vi "run_experiment_sCMOS_DAC.vi"() -> ()   [LabVIEW 2015]
uses:
  <vilib>/DAQmx/write.llb/DAQmx Write (Digital Bool 1Line 1Point).vi
  <vilib>/DAQmx/read.llb/DAQmx Read (Analog 1D Wfm NChan NSamp).vi
  <vilib>/DAQmx/read.llb/DAQmx Read (Digital 2D U32 NChan NSamp).vi
  <vilib>/DAQmx/write.llb/DAQmx Write (Digital 1D Wfm NChan NSamp).vi
  <vilib>/DAQmx/write.llb/DAQmx Write (Analog 1D DBL 1Chan NSamp).vi
  <vilib>/DAQmx/create/channels.llb/DAQmx Create Channel (DO-Digital Output).vi
  <vilib>/DAQmx/miscellaneous.llb/DAQmx Fill In Error Info.vi
  <vilib>/Utility/file.llb/Write Delimited Spreadsheet (DBL).vi
  <vilib>/Waveform/DWDTOps.llb/DWDT Uncompress Digital.vi
  <vilib>/addons/h5labview2/file/H5F.lvlib
panel:
  in  "New Session?":bool
  in  "New Session Type":enum32{"recording", "roi", "rig_state"}(radio)
  in  "Use Cam":bool
  in  "Pad Stim":bool
  out "Timestamp":string
  out "Genotype":string
  out "Fly Name":string
  out "Experiment Name":string
  out ".dcimg index":i32
  out ".dcimg count":i32
  in  "Use .dcimg":bool
  out "Cumulative Frames":i32
  out "N Stim Frames":i32
  out "Trial":i32
  out "N Samps 2 Write":i32
  out "AI/DI SampRate":dbl=1000.0 format="%0.2f"
  out "AO/DO SampRate":dbl
  out "DO Samps Written":u32
  out "AO Samps Written":u32
  out "Protocol Rate (Hz)":i32
  out "Num Stimuli":i32
  out "V Offset":i32
  out "H Offset":i32
  out "Rep":i32
  out ".dcimg --> .tiff":bool
  out "# tiffs":i32
  in  "Save .tiffs":bool
  in  "Configure Cam":bool
  out "Stimulus Order":i32[](array[numeric])
  in  "Randomize":bool
  out "Stop Input":bool
  out "temp .dcimg filepath":path
  out "Exposure":dbl
  out "V Width":i32
  out "H Width":i32
  out "Acquiring Frames":bool
  out "Current Stim Duration":dbl
  out "Current Stimulus Save Path":path
  in  "N Reps":dbl
  out "Experiment Path":path
  in  "Metadata Path":path
  out "Stimulus Files":path[](array[path])
  out "Protocol Name":string
  in  "Protocol Path":path
  out "Display":T1(plugin-control)
  out "DAC Input":waveform(dbl)[](graph) caption="DAC Input Display"
  out "error out":errorcluster
  out "Current Stimulus Name":string
  out "Curr Piezo Cmd":waveform(dbl)(graph)
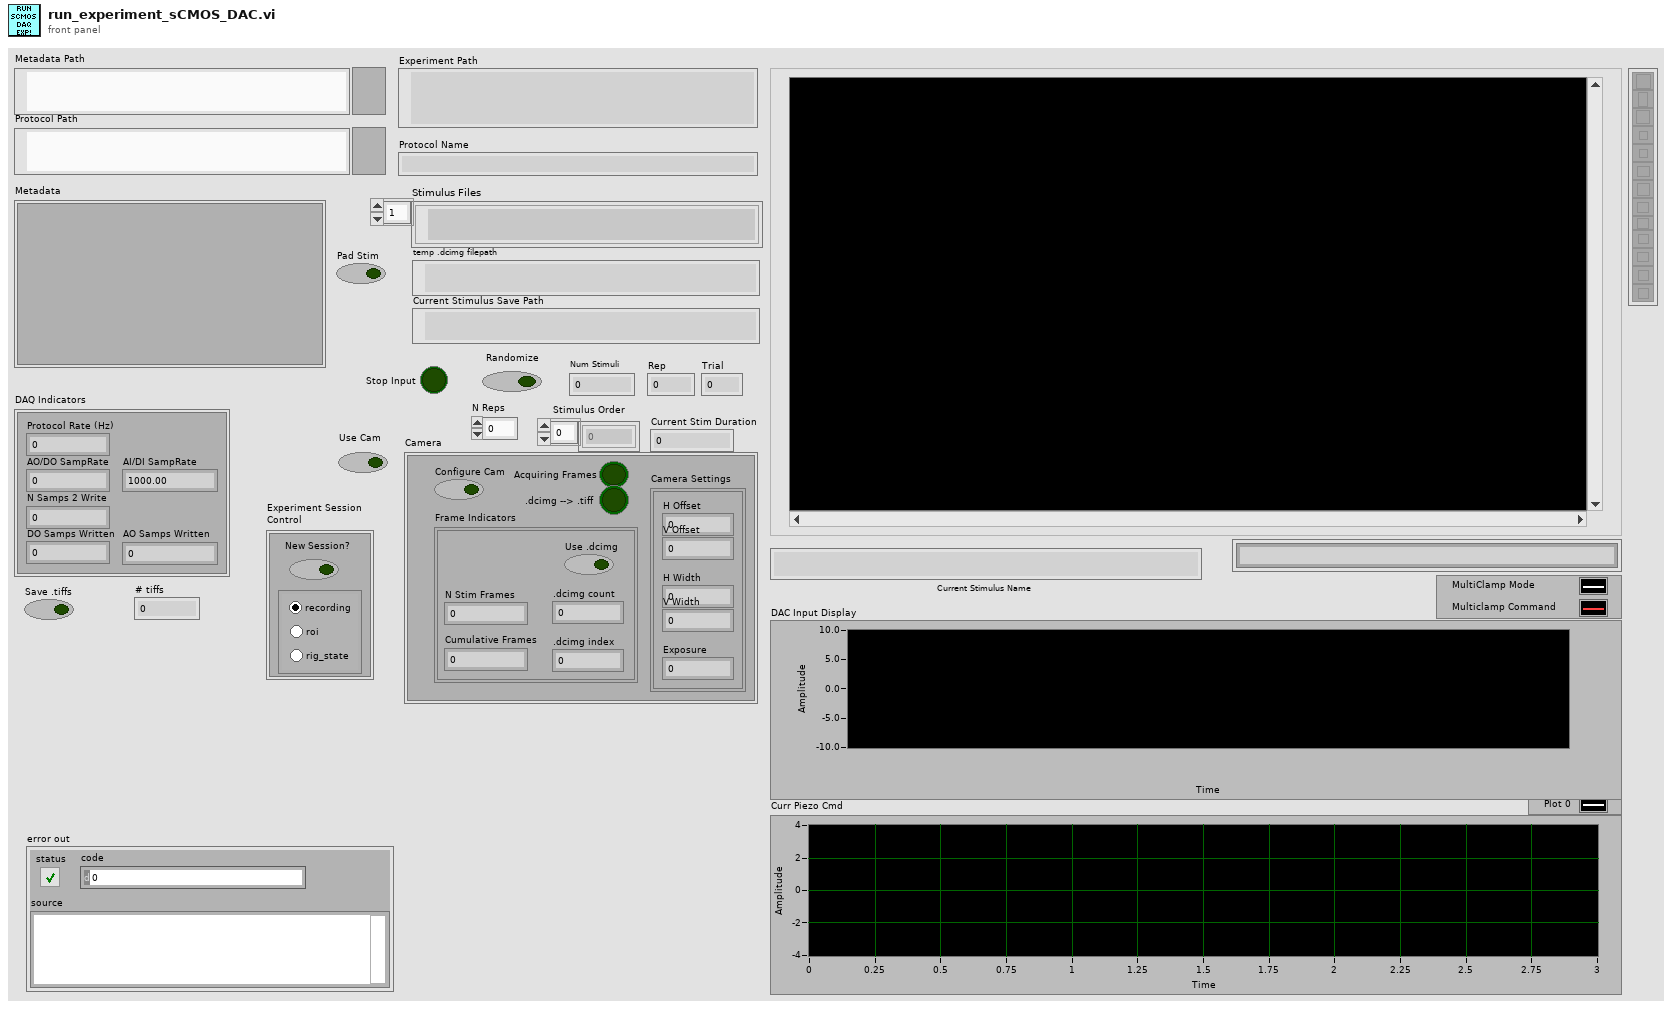
[diagram p1: front panel]
types:
  T1 = typedef "IMAQ Image.ctl" = refnum<image>
  T2 = cluster{"Value":i32, "Minimum":i32, "Maximum":i32, "Increment":i32}
  T3 = cluster{"Rows Per Strip":i32, "Photometric":i32, "Compression Type":i32}
  T4 = cluster{"piezo_command":dbl[], "alignment_command":dbl[]}
  T5 = typedef "Image Type" = u32
  T6 = cluster{"height":u32, "width":u32, "datatype":u32}
  T7 = cluster{"piezo_cmd":i32, "piezo_sensor":i32, "cam_trig_1":i32, "cam_trig_2":i32, "alignment_cmd":i32, "mc700b_primary":i32, "mc700b_secondary":i32, "mc700b_mode":i32, "mc700b_cmd":i32}
  T8 = typedef "hid_t.ctl" = i32
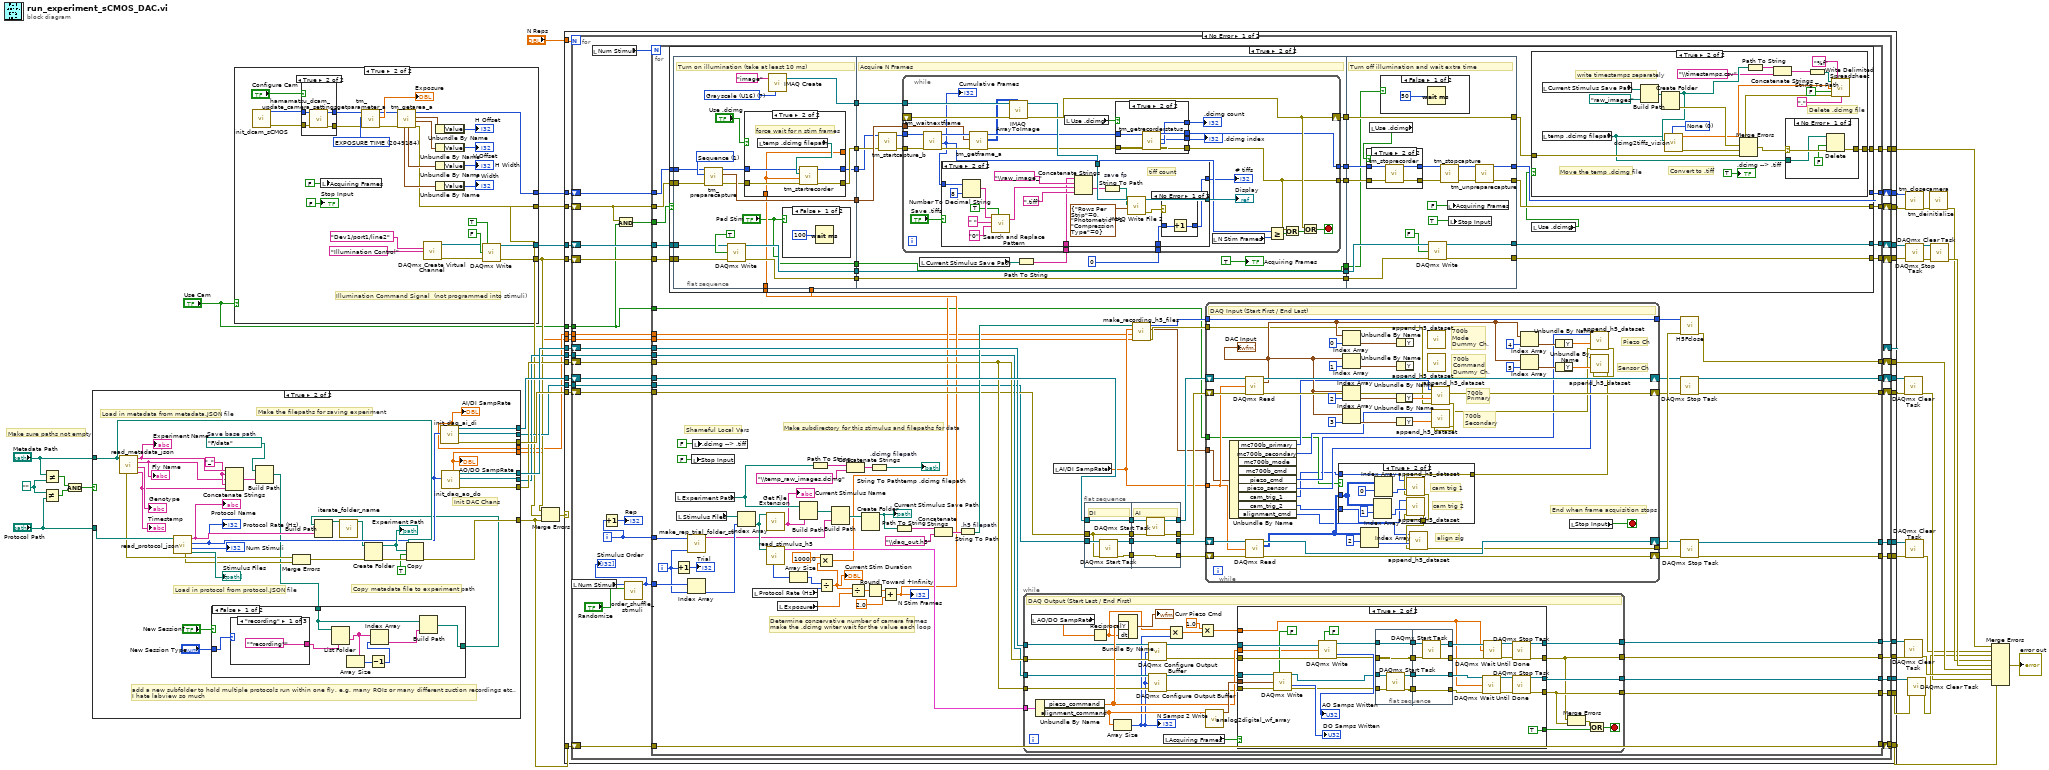
[diagram p0: block diagram]
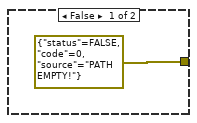
[diagram p4: hidden frame]
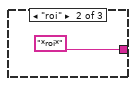
[diagram p5: hidden frame]
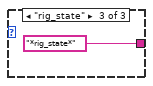
[diagram p6: hidden frame]
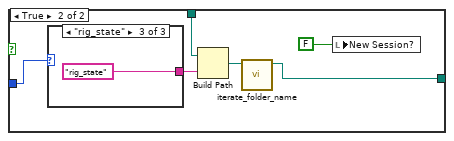
[diagram p7: hidden frame]
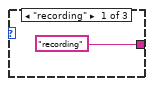
[diagram p8: hidden frame]
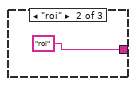
[diagram p9: hidden frame]
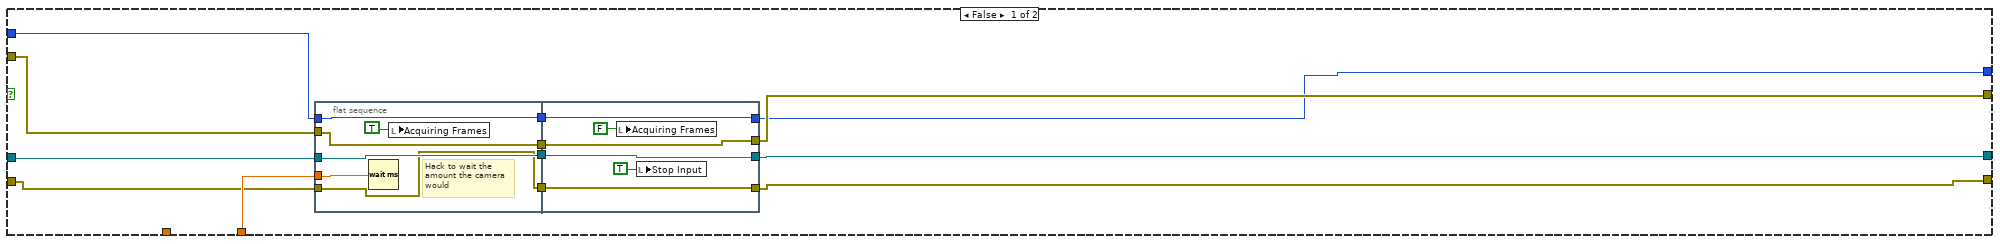
[diagram p10: hidden frame]
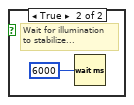
[diagram p13: hidden frame]
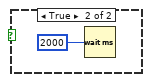
[diagram p18: hidden frame]
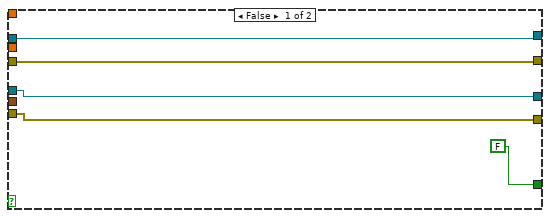
[diagram p20: hidden frame]
diagram:
  w11 = path ""
  # "Make sure paths not empty"
  n1 = Not Equal?(x=w11, y="Protocol Path") -> (x != y?=w13:bool)
  n2 = Not Equal?(x="Metadata Path", y=w11) -> (x != y?=w14:bool)
  n3 = And(x=w14, y=w13) -> (x .and. y?=w23:bool)
  n4 = case shown="True" w23 {
    tunnel: [errorcluster {"status"=FALSE, "code"=0, "source"="PATH EMPTY!"} ("error out") w82] -> w7
    tunnel: "Metadata Path" -> [_ w81]
    tunnel: "Protocol Path" -> [_ w80]
    tunnel: [_ w79] -> w27
    tunnel: [_ w78] -> w26
    tunnel: [_ w77] -> w25
    tunnel: [_ w76] -> w24
    tunnel: [_ w75] -> w22
    tunnel: [_ w74] -> w8
    tunnel: [_ w56] -> w2
    tunnel: [_ w55] -> w1
    frame False {
    }
    frame True {
      w61 = "_"
      w70 = path "F:/data"  # Save base path
      # "add a new subfolder to hold multiple protocols run within one fly, e.g. many ROIs or many different suction recordings etc.,\nI hate labview so much"
      # "Init DAC Chans"
      # "Load in metadata from metadata.JSON file"
      # "Load in protocol from protocol.JSON file"
      # "Copy metadata file to experiment path"
      # "Make the filepaths for saving experiment"
      n5 = call "read_metadata_json.vi"("Path"=w81) -> ("exp_time"=w62:string, "genotype"=→"Genotype":string, "fly_name"=w60:string, "exp_ name"=w66:string, "error out"=w65:errorcluster)  [unwired: 6 in]
      "Experiment Name" <- w66
      "Fly Name" <- w60
      "Timestamp" <- w62
      n6 = call "read_protocol_json.vi"("Path"=w80) -> ("stims"=→"Stimulus Files":path[], "n_stims"=→"Num Stimuli":i32, "rate"=w57:i32, "protocol name"=w59:string, "error out"=w64:errorcluster)  [unwired: 6 in]
      "Protocol Rate (Hz)" <- w57
      "Protocol Name" <- w59
      n7 = Concatenate Strings(w66, w61, w60, w61, w62) -> (w58:string)
      n8 = Build Path(base path=w70, name or relative path=w58) -> (appended path=w49:path)
      n9 = case shown="False" "New Session?" {
        tunnel: "New Session Type" -> [w90 w94]
        tunnel: [w84 w97] -> w50
        tunnel: w49 -> [w85 w95]
        frame False {
          n10 = case shown="\"recording\"" w90 {
            tunnel: ["*recording*" "*roi*" "*rig_state*"] -> w83
            frame "recording" {
            }
            frame "roi" {
            }
            frame "rig_state" {
            }
          }
          n11 = List Folder(path=w85, pattern=w83) -> (folder names=w89:string[])  [unwired: 2 in, 3 out]
          n12 = Array Size(array=w89) -> (size(s)=w88:i32)
          n13 = Decrement(x=w88) -> (x-1=w87:i32)
          n14 = Index Array(array=w89, index=w87) -> (element=w86:string)
          n15 = Build Path(base path=w85, name or relative path=w86) -> (appended path=w84:path)
        }
        frame True {
          n16 = case shown="\"rig_state\"" w94 {
            tunnel: ["recording" "roi" "rig_state"] -> w96
            frame "recording" {
            }
            frame "roi" {
            }
            frame "rig_state" {
            }
          }
          n17 = Build Path(base path=w95, name or relative path=w96) -> (appended path=w98:path)
          n18 = call "iterate_folder_name.vi"("Folder In"=w98) -> ("Folder Out"=w97:path)  [unwired: 10 in]
          n19 = local write "New Session?"(FALSE ("Boolean")) -> ()
        }
      }
      n20 = Merge Errors(w65, w64) -> (w63:errorcluster)
      n21 = Build Path(base path=w50, name or relative path=w59) -> (appended path=w54:path)
      n22 = call "iterate_folder_name.vi"("Folder In"=w54) -> ("Folder Out"=w53:path)  [unwired: 10 in]
      n23 = Create Folder(path (use dialog)=w53, error in=w63) -> (created path=w73:path, error out=w72:errorcluster)  [unwired: 1 in, 1 out]
      "Experiment Path" <- w73
      n24 = Copy(8:w72, 9:TRUE ("overwrite (F)"), 10:w73, 11:w81) -> (0:w82:errorcluster)  [unwired: 1 in, 2 out]
      n25 = call "init_daq_ai_di.vi"("Sample Rate"=w57) -> ("error out"=w78:errorcluster, "DI Out"=w74:refnum<k21>, "AI Out"=w79:refnum<k21>, "Actual Sample Rate"=w56:dbl)  [unwired: 7 in]
      "AI/DI SampRate" <- w56
      n26 = call "init_daq_ao_do.vi"("Rate"=w57) -> ("error out"=w76:errorcluster, "DO Out"=w75:refnum<k21>, "AO Out"=w77:refnum<k21>, "AO SampClk.Rate"=w55:dbl)  [unwired: 7 in]
      "AO/DO SampRate" <- w55
    }
  }
  n27 = case shown="True" "Use Cam" {
    tunnel: [_ w128] -> w31
    tunnel: [_ w126] -> w30
    tunnel: [_ w104] -> w6
    tunnel: [_ w103] -> w4
    frame False {
    }
    frame True {
      w121 = u32 2049184 items=["SENSOR MODE"=4212128, "CCD MODE"=4212384, "READOUT MODE"=4211872, "ACTIVE VIEW INDEX"=4343136, "BITS PER CHANNEL"=4342976, "IMAGE PIXEL TYPE"=4343296, "BINNING"=4215968, "EXPOSURE TIME"=2049184, "CONTRAST GAIN"=3163312, "CONTRAST OFFSET"=3163328, "LIGHT MODE"=2114720, "SENSITIVITY"=2114992, "PHOTON IMAGING MODE"=2115200, "HIGH DYNAMIC RANGE MODE"=3163360, "WHITE BALANCE"=3163568, "TEMPERATURE"=2115232, "TEMPERATURE TARGET"=2115264, "SENSOR COOLER FAN"=2115296, "LINEBUNDLE HEIGHT"=4212192, "MECHANICAL SHUTTER"=2115488, "BACK FOCUS POSITION"=8422304, "TRIGGER CONNECTOR"=1066432, "TRIGGER SOURCE"=1066144, "OUTPUT TRIGGER SOURCE"=1852576, "TRIGGER GLOBAL EXPOSURE"=2049680, "FIRST TRIGGER BEHAVIOR"=2049696, "CHANNEL SYNC"=1852352, "READOUT DIRECTION"=4211904, "PRE HSYNC COUNT"=1852704] ("Parameter")
      # "Illumination Command Signal  (not programmed into stimuli)"
      n28 = call "init_dcam_sCMOS.vi"() -> ("error out"=w106:errorcluster, "Handle out"=w107:u32)  [unwired: 10 in]
      n29 = case shown="True" "Configure Cam" {
        tunnel: [w132 w137] -> w112
        tunnel: [w133 w136] -> w111
        tunnel: w107 -> [w133 w135]
        tunnel: w106 -> [w132 w134]
        frame False {
        }
        frame True {
          n30 = call "hamamatsu_dcam_update_camera_settings.vi"("error in (no error)"=w134, "Handle in"=w135) -> ("error out"=w137:errorcluster, "Handle out"=w136:u32)  [unwired: 6 in]
        }
      }
      n31 = local write "Acquiring Frames"(FALSE ("Acquiring Frames")) -> ()
      n32 = call <userlib>:"tm_getparameter_a.vi"("error in (no error)"=w112, "Parameter"=w121, "Handle in"=w111) -> ("error out"=w116:errorcluster, "Value out"=→"Exposure":dbl, "Handle out"=w115:u32)  [unwired: 6 in]
      n33 = call <userlib>:"tm_getarea_a.vi"("error in (no error)"=w116, "Handle in"=w115) -> ("error out"=w104:errorcluster, "V Offset"=w119:T2, "H Offset"=w120:T2, "Handle out"=w126:u32, "H Width"=w118:T2, "V Width"=w117:T2)  [unwired: 4 in]
      n34 = call-poly <vilib>:"DAQmx Create Virtual Channel.vi"("lines"=tag "Dev1/port1/line2", "name to assign"="Illumination Control") -> ("task out"=w124:refnum<k21>, "error out"=w123:errorcluster)  [unwired: 12 in]
      n35 = Unbundle By Name(w120) -> ("Value"=→"H Offset":i32)
      n36 = Unbundle By Name(w119) -> ("Value"=→"V Offset":i32)
      n37 = Unbundle By Name(w118) -> ("Value"=→"H Width":i32)
      n38 = Unbundle By Name(w117) -> ("Value"=→"V Width":i32)
      n39 = call-poly <vilib>:"DAQmx Write.vi"("task/channels in"=w124, "auto start"=TRUE, "data"=FALSE, "error in"=w123) -> ("task out"=w128:refnum<k21>, "error out"=w103:errorcluster)  [unwired: 9 in, 1 out]
      "Stop Input" <- FALSE ("Stop Input")
    }
  }
  n40 = Merge Errors(w4, w6, w7) -> (w5:errorcluster)
  n41 = case shown="No Error" w5 {
    tunnel: w30 -> [w167 w639]
    tunnel: w6 -> [w166 w638]
    tunnel: [w160 _] -> w39
    tunnel: [w159 _] -> w40
    tunnel: [w165 _] -> w9
    tunnel: [w164 _] -> w43
    tunnel: [w163 w638] -> w36
    tunnel: [w162 w639] -> w35
    tunnel: [w161 _] -> w42
    tunnel: [w158 _] -> w34
    tunnel: [w157 _] -> w33
    tunnel: w31 -> [w156 _]
    tunnel: w4 -> [w155 _]
    tunnel: w27 -> [w154 _]
    tunnel: w26 -> [w153 _]
    tunnel: w25 -> [w152 _]
    tunnel: w24 -> [w151 _]
    tunnel: [w150 _] -> w15
    tunnel: w7 -> [w149 _]
    tunnel: [w148 _] -> w29
    tunnel: w22 -> [w147 _]
    tunnel: [w146 _] -> w19
    tunnel: [w145 _] -> w20
    tunnel: [w144 _] -> w18
    tunnel: [w143 _] -> w17
    tunnel: "N Reps" -> [w142 _]
    tunnel: w8 -> [w141 _]
    tunnel: "Use Cam" -> [w140 _]
    tunnel: w2 -> [w139 _]
    tunnel: w1 -> [w138 _]
    frame No Error {
      n42 = for {
        N: w142 -> [_]
        tunnel: [w187] -> w150
        tunnel: [w185] -> w148
        shift-right: [w199] -> w162
        shift-left: w167 -> [w203]
        shift-right: [w200] -> w163
        shift-left: w166 -> [w172]
        shift-right: [w197] -> w160
        shift-left: w156 -> [w193]
        shift-right: [w196] -> w159
        shift-left: w155 -> [w192]
        shift-right: [w194] -> w157
        shift-left: w154 -> [w191]
        shift-right: [w195] -> w158
        shift-left: w153 -> [w190]
        shift-right: [w201] -> w164
        shift-left: w152 -> [w189]
        shift-right: [w198] -> w161
        shift-left: w151 -> [w188]
        shift-right: [w202] -> w165
        shift-left: w149 -> [w186]
        tunnel: w147 -> [w184]
        tunnel: [w183] -> w146
        tunnel: [w182] -> w145
        tunnel: [w181] -> w144
        tunnel: [w180] -> w143
        tunnel: w141 -> [w175]
        tunnel: w140 -> [w168]
        tunnel: w139 -> [w170]
        tunnel: w138 -> [w169]
        i -> [w173]
        n43 = local read "Num Stimuli"() -> (w178:i32)
        n44 = local read "Num Stimuli"() -> (w177:i32)
        n45 = Increment(x=w173) -> (x+1=→"Rep":i32)
        n46 = And(x=w172, y=w168) -> (x .and. y?=w171:bool)
        n47 = call "order_shuffle_stimuli.vi"("Randomize?"="Randomize", "N Stimuli"=w178) -> ("Riffled"=w176:i32[])  [unwired: 9 in]
        "Stimulus Order" <- w176
        n48 = for {
          N: w177 -> [_]
          tunnel: w203 -> [w267]
          tunnel: w172 -> [w221]
          tunnel: [w281] -> w202
          tunnel: [w280] -> w201
          tunnel: [w253] -> w200
          tunnel: [w254] -> w199
          tunnel: [w276] -> w198
          tunnel: [w273] -> w197
          tunnel: [w272] -> w196
          tunnel: [w271] -> w195
          tunnel: [w270] -> w194
          tunnel: w193 -> [w255]
          tunnel: w192 -> [w256]
          tunnel: w191 -> [w269]
          tunnel: w190 -> [w232]
          tunnel: w189 -> [w268]
          tunnel: w188 -> [w238]
          tunnel: [w249] -> w187
          tunnel: w186 -> [w248]
          tunnel: [w248] -> w185
          tunnel: w176 -> [w240]
          tunnel: w173 -> [w217]
          tunnel: w184 -> [w237]
          tunnel: [w236] -> w183
          tunnel: [w235] -> w182
          tunnel: [w225] -> w181
          tunnel: [w224] -> w180
          tunnel: w175 -> [w214]
          tunnel: w171 -> [w210]
          tunnel: w170 -> [w206]
          tunnel: w169 -> [w205]
          tunnel: w168 -> [w204]
          i -> [w212]
          # "Shameful Local Vars"
          # "Determine conservative number of camera frames\nmake the .dcimg writer wait for the value each loop"
          # "Make subdirectory for this stimulus and filepaths for data"
          n49 = Increment(x=w212) -> (x+1=→"Trial":i32)
          n50 = local read "Experiment Path"() -> (w258:path)
          n51 = local read "Stimulus Files"() -> (w285:path[])
          n52 = Index Array(array=w240, index=w212) -> (element=w241:i32)
          n53 = call "make_rep_trial_folder_str.vi"("trial"=w212, "rep"=w217) -> ("folder string"=w216:string)  [unwired: 6 in]
          n54 = local write "Stop Input"(FALSE ("Stop Input")) -> ()
          n55 = local write ".dcimg --> .tiff"(FALSE ("Converting .tiff")) -> ()
          n56 = Index Array(array=w285, index=w241) -> (element=w220:path)
          n57 = local read "Protocol Rate (Hz)"() -> (w250:i32)
          n58 = call <vilib>:"Get File Extension.vi"("file"=w220) -> ("filename without extension"=w243:string)  [unwired: 6 in, 4 out]
          "Current Stimulus Name" <- w243
          n59 = call "read_stimulus_h5.vi"("Path"=w220) -> ("output cluster"=w223:T4, "piezo_command"=w222:i32[])  [unwired: 7 in, 2 out]
          n60 = local read "Exposure"() -> (w218:dbl)
          n61 = Array Size(array=w222) -> (size(s)=w251:i32)
          n62 = Build Path(base path=w258, name or relative path=w243) -> (appended path=w262:path)
          n63 = Path To String(path=w258) -> (string=w264:string)
          n64 = Divide(x=w251, y=w250) -> (x/y=w209:dbl)
          "Current Stim Duration" <- w209
          n65 = Multiply(x=1000.0, y=w209) -> (x*y=w207:dbl)
          n66 = Build Path(base path=w262, name or relative path=w216) -> (appended path=w263:path)
          n67 = Concatenate Strings(w264, "\\temp_raw_images.dcimg" ("string")) -> (w266:string)
          n68 = Divide(x=w209, y=w218) -> (x/y=w284:dbl)
          n69 = Create Folder(path (use dialog)=w263) -> (created path=w252:path)  [unwired: 2 in, 2 out]
          "Current Stimulus Save Path" <- w252
          n70 = Round Toward +Infinity(x=w284) -> (ceil(x): smallest int >= x=w283:dbl)
          n71 = String To Path ".dcimg filepath"(string=w266) -> (path=→"temp .dcimg filepath":path)
          n72 = Add(x=w283, y=2.0) -> (x+y=w213:dbl)
          "N Stim Frames" <- w213
          n73 = case shown="True" w210 {
            tunnel: [w300 w332] -> w273
            tunnel: [w297 w331] -> w272
            tunnel: w267 -> [w305 w341]
            tunnel: w221 -> [w308 w340]
            tunnel: w256 -> [w299 w339]
            tunnel: w255 -> [w302 w338]
            tunnel: [w303 w337] -> w254
            tunnel: [w306 w336] -> w253
            tunnel: [_ w334] -> w249
            tunnel: w213 -> [_ w326]
            tunnel: w207 -> [w309 _]
            frame False {
              n74 = flat-sequence {
                tunnel: w309 -> [w314]
                tunnel: w308 -> [w313]
                tunnel: [w313] -> w307
                tunnel: w305 -> [w312]
                tunnel: [w312] -> w304
                tunnel: w302 -> [w311]
                tunnel: [w311] -> w301
                tunnel: w299 -> [w310]
                tunnel: [w310] -> w298
                tunnel: [w320] -> w306
                tunnel: w307 -> [w320]
                tunnel: [w319] -> w303
                tunnel: w304 -> [w319]
                tunnel: [w318] -> w300
                tunnel: w301 -> [w318]
                tunnel: [w317] -> w297
                tunnel: w298 -> [w317]
                frame #0 {
                  # "Hack to wait the \namount the camera\nwould"
                  n75 = Wait (ms)(milliseconds to wait=w314) -> ()  [unwired: 1 out]
                  n76 = local write "Acquiring Frames"(TRUE ("Acquiring Frames")) -> ()
                }
                frame #1 {
                  n77 = local write "Acquiring Frames"(FALSE) -> ()
                  n78 = local write "Stop Input"(TRUE ("Stop Input")) -> ()
                }
              }
            }
            frame True {
              n79 = flat-sequence {
                tunnel: [w389] -> w346
                tunnel: [w386] -> w345
                tunnel: w341 -> [w391]
                tunnel: w340 -> [w390]
                tunnel: w339 -> [w384]
                tunnel: w338 -> [w383]
                tunnel: [w379] -> w330
                tunnel: [w378] -> w327
                tunnel: w326 -> [w377]
                tunnel: [w376] -> w325
                tunnel: [w375] -> w324
                tunnel: ["Pad Stim"] -> w322
                tunnel: w346 -> [w418]
                tunnel: [w413] -> w344
                tunnel: [w417] -> w343
                tunnel: w345 -> [w416]
                tunnel: [w415] -> w342
                tunnel: w330 -> [w412]
                tunnel: [w412] -> w329
                tunnel: [w411] -> w328
                tunnel: w327 -> [w411]
                tunnel: w325 -> [w406]
                tunnel: w324 -> [w405]
                tunnel: [w404] -> w323
                tunnel: w322 -> [w404]
                tunnel: w344 -> [w486]
                tunnel: w343 -> [w487]
                tunnel: [w491] -> w336
                tunnel: [w493] -> w337
                tunnel: w342 -> [w495]
                tunnel: [w495] -> w335
                tunnel: [w484] -> w332
                tunnel: [w483] -> w331
                tunnel: w329 -> [w481]
                tunnel: w328 -> [w480]
                tunnel: w323 -> [w478]
                frame #0 {
                  w388 = T5 7 items=["Grayscale (U8)", "Grayscale (I16)", "Grayscale (SGL)", "Complex (CSG)", "RGB (U32)", "HSL (U32)", "RGB (U64)", "Grayscale (U16)"] ("Image Type")
                  w392 = 1 items=["Snap", "Sequence"] ("Capture mode")
                  # "Turn on illumination (take at least 10 ms)"
                  n80 = call <userlib>:"tm_preparecapture.vi"("error in (no error)"=w390, "Capture mode"=w392, "Handle in"=w391) -> ("error out"=w381:errorcluster, "Buffer Info"=w389:T6, "Handle out"=w380:u32)  [unwired: 5 in, 1 out]
                  n81 = call-poly <vilib>:"DAQmx Write.vi"("task/channels in"=w383, "data"=TRUE, "error in"=w384) -> ("task out"=w378:refnum<k21>, "error out"=w379:errorcluster)  [unwired: 10 in, 1 out]
                  n82 = case shown="True" "Use .dcimg" {
                    tunnel: [w397 w402] -> w375
                    tunnel: [w396 w401] -> w376
                    tunnel: w381 -> [w396 w400]
                    tunnel: w380 -> [w397 w399]
                    tunnel: w377 -> [w395 w398]
                    tunnel: [w395 w398] -> _
                    frame False {
                      # "still force waiting on\nstim frame calculation"
                    }
                    frame True {
                      # "force wait for n stim frames"
                      n83 = local read "temp .dcimg filepath"() -> (w403:path)
                      n84 = call <userlib>:"tm_startrecorder.vi"("error in (no error)"=w400, "frames"=w398, "File"=w403, "Handle in"=w399) -> ("error out"=w401:errorcluster, "Handle out"=w402:u32)  [unwired: 6 in]
                    }
                  }
                  n85 = call "IMAQ Create"("Image Name"="image", "Image Type"=w388) -> ("New Image"=w386:T1)  [unwired: 3 in, 1 out]
                  n86 = case shown="False" "Pad Stim" {
                    frame False {
                      n87 = Wait (ms)(milliseconds to wait=u32 100) -> ()  [unwired: 1 out]
                    }
                    frame True {
                      # "Wait for illumination\nto stabilize..."
                      n88 = Wait (ms)(milliseconds to wait=u32 6000) -> ()  [unwired: 1 out]
                    }
                  }
                }
                frame #1 {
                  # "Acquire N Frames"
                  n89 = call <userlib>:"tm_startcapture_b.vi"("error in (no error)"=w406, "Handle in"=w405) -> ("error out"=w407:errorcluster, "Handle out"=w408:u32)  [unwired: 8 in]
                  n90 = local read "Current Stimulus Save Path"() -> (w414:path)
                  n91 = Path To String(path=w414) -> (string=w410:string)
                  n92 = while {
                    tunnel: w407 -> [w444]
                    tunnel: w418 -> [w443]
                    tunnel: w408 -> [w442]
                    tunnel: [w428] -> w413
                    tunnel: [w423] -> w417
                    tunnel: w416 -> [w440]
                    shift-right: [w437] -> w415
                    shift-left: _ -> [w439]
                    tunnel: w410 -> [w426]
                    tunnel: 0 -> [w421]
                    stop <- w435 stop-if-true
                    n93 = call <userlib>:"tm_waitnextframe.vi"("error in (no error)"=w444, "Handle in"=w442) -> ("error out"=w446:errorcluster, "Frame Count"=w425:i32, "Handle out"=w445:u32)  [unwired: 6 in, 1 out]
                    "Cumulative Frames" <- w425
                    n94 = call <userlib>:"tm_getframe_a.vi"("error in (no error)"=w446, "Buffer Info"=w443, "Handle in"=w445) -> ("error out"=w430:errorcluster, "Data 16"=w427:u16[][], "Handle out"=w429:u32)  [unwired: 4 in, 2 out]
                    n95 = call "IMAQ ArrayToImage"("Image Pixels (U16)"=w427, "error in (no error)"=w439, "Image"=w440) -> ("error out"=w437:errorcluster, "Image Out"=w434:T1)  [unwired: 7 in]
                    n96 = case shown="True" "Save .tiffs" {
                      tunnel: w434 -> [w456 w474]
                      tunnel: [w456 w472] -> w433
                      tunnel: w426 -> [_ w460]
                      tunnel: w425 -> [_ w461]
                      tunnel: [w455 w458] -> w422
                      tunnel: w421 -> [w455 w459]
                      frame False {
                      }
                      frame True {
                        # "tiff count"
                        n97 = Number To Decimal String(number=w461, width (-)=i16 8) -> (decimal integer string=w470:string)
                        n98 = call <vilib>:"Search and Replace Pattern.vi"("string"=w470, "regular expression (\"\")"=" " ("regular expression (\"\")"), "replace string (\"\")"="0" ("replace string (\"\")"), "replace all? (F)"=TRUE) -> ("result string"=w471:string)  [unwired: 1 in, 1 out]
                        n99 = Concatenate Strings(w460, "\\raw_image_" ("string"), w471, ".tiff" ("string")) -> (w464:string)
                        n100 = String To Path "save fp"(string=w464) -> (path=w462:path)
                        n101 = call-poly "IMAQ Write File 2"("TIFF Options"=T3 {"Rows Per Strip"=0, "Photometric"=1, "Compression Type"=0}, "File Path"=w462, "Image"=w474) -> ("error out"=w457:errorcluster, "Image Out (duplicate)"=w472:T1)  [unwired: 7 in]
                        n102 = case shown="No Error" w457 {
                          tunnel: w459 -> [w476 w477]
                          tunnel: [w475 w477] -> w458
                          frame No Error {
                            n103 = Increment(x=w476) -> (x+1=w475:i32)
                          }
                          frame Error {
                          }
                        }
                      }
                    }
                    "Display" <- w433
                    "# tiffs" <- w422
                    n104 = local read "Use .dcimg"() -> (w431:bool)
                    n105 = case shown="True" w431 {
                      tunnel: w430 -> [w448 w454]
                      tunnel: [w448 w453] -> w423
                      tunnel: w429 -> [w447 w452]
                      tunnel: [w447 w451] -> w428
                      tunnel: [_ w450] -> w424
                      tunnel: [_ w449] -> w420
                      frame False {
                      }
                      frame True {
                        n106 = call <userlib>:"tm_getrecorderstatus.vi"("error in (no error)"=w454, "Handle"=w452) -> ("error out"=w453:errorcluster, "Count"=w450:i32, "Index"=w449:i32, "Handle"=w451:u32)  [unwired: 6 in]
                      }
                    }
                    ".dcimg count" <- w424
                    ".dcimg index" <- w420
                    n107 = local read "N Stim Frames"() -> (w441:i32)
                    n108 = Greater Or Equal?(x=w425, y=w441) -> (x >= y?=w438:bool)
                    n109 = Or(x=w423, y=w438) -> (x .or. y?=w436:bool)
                    n110 = Or(x=w437, y=w436) -> (x .or. y?=w435:bool)
                  }
                  "Acquiring Frames" <- TRUE
                }
                frame #2 {
                  # "Turn off illumination and wait extra time"
                  n111 = local read "Use .dcimg"() -> (w489:bool)
                  n112 = case shown="True" w489 {
                    tunnel: [w499 w502] -> w488
                    tunnel: w487 -> [w499 w503]
                    tunnel: w486 -> [w498 w500]
                    tunnel: [w498 w501] -> w485
                    frame False {
                    }
                    frame True {
                      n113 = call <userlib>:"tm_stoprecorder.vi"("error in (no error)"=w503, "Handle in"=w500) -> ("error out"=w502:errorcluster, "Handle out"=w501:u32)  [unwired: 8 in]
                    }
                  }
                  n114 = case shown="False" w478 {
                    frame False {
                      n115 = Wait (ms)(milliseconds to wait=50 ("ms between stimuli")) -> ()  [unwired: 1 out]
                    }
                    frame True {
                      n116 = Wait (ms)(milliseconds to wait=2000 ("ms between stimuli")) -> ()  [unwired: 1 out]
                    }
                  }
                  n117 = call-poly <vilib>:"DAQmx Write.vi"("task/channels in"=w480, "data"=FALSE, "error in"=w481) -> ("task out"=w484:refnum<k21>, "error out"=w483:errorcluster)  [unwired: 10 in, 1 out]
                  n118 = call <userlib>:"tm_stopcapture.vi"("error in (no error)"=w488, "Handle in"=w485) -> ("error out"=w492:errorcluster, "Handle out"=w494:u32)  [unwired: 8 in]
                  n119 = local write "Acquiring Frames"(FALSE) -> ()
                  n120 = local write "Stop Input"(TRUE ("Stop Input")) -> ()
                  n121 = call <userlib>:"tm_unpreparecapture.vi"("error in (no error)"=w492, "Handle in"=w494) -> ("error out"=w491:errorcluster, "Handle out"=w493:u32)  [unwired: 8 in]
                }
              }
              n122 = local read "Use .dcimg"() -> (w333:bool)
              n123 = case shown="True" w333 {
                tunnel: w335 -> [w347 w359]
                tunnel: [w347 w360] -> w334
                frame False {
                }
                frame True {
                  w364 = 0 items=["None", "JPEG", "Run Length Encoded", "Zip"] ("Compression Type")
                  # "write timestamps separately"
                  # "Delete .dcimg file"
                  # "Convert to .tiff"
                  # "Move the temp .dcimg file"
                  n124 = local read "Current Stimulus Save Path"() -> (w367:path)
                  n125 = local read "temp .dcimg filepath"() -> (w348:path)
                  n126 = Build Path(base path=w367, name or relative path=path "raw_images") -> (appended path=w365:path)
                  n127 = Create Folder(path (use dialog)=w365) -> (created path=w358:path, error out=w363:errorcluster)  [unwired: 2 in, 1 out]
                  n128 = call "dcimg2tiffs_vision.vi"("Compression Type"=w364, ".tiff Path"=w358, "DCIMG Path"=w348) -> ("Error Out"=w368:errorcluster, "Timestamps"=w353:dbl[])  [unwired: 7 in]
                  n129 = Path To String(path=w358) -> (string=w357:string)
                  n130 = Concatenate Strings(w357, "\\timestamps.csv" ("string")) -> (w355:string)
                  n131 = String To Path(string=w355) -> (path=w354:path)
                  n132 = call-poly <vilib>:"Write Delimited Spreadsheet.vi"("file path (dialog if empty)"=w354, "format (%.3f)"="%f", "1D data"=w353, "append to file? (F)"=FALSE, "delimiter (\\t)"="," ("delimiter (\\t)")) -> ("error out"=w352:errorcluster)  [unwired: 9 in, 1 out]
                  n133 = Merge Errors(w352, w363, w368, w359) -> (w361:errorcluster)
                  n134 = case shown="No Error" w361 {
                    selector: w361 -> [w372 w373]
                    tunnel: [w371 w373] -> w360
                    tunnel: w348 -> [w369 _]
                    frame No Error {
                      n135 = Delete(path (use dialog)=w369, confirm (F)=FALSE, error in=w372) -> (error out=w371:errorcluster)  [unwired: 2 in, 2 out]
                    }
                    frame Error {
                    }
                  }
                  ".dcimg --> .tiff" <- TRUE ("Converting .tiff")
                }
              }
            }
          }
          n136 = Path To String(path=w252) -> (string=w260:string)
          n137 = Concatenate Strings(w260, "\\daq_out.h5" ("string")) -> (w259:string)
          n138 = String To Path ".h5 filepath"(string=w259) -> (path=w247:path)
          n139 = while {
            tunnel: w268 -> [w511]
            tunnel: [w529] -> w280
            tunnel: [w525] -> w281
            tunnel: w238 -> [w510]
            tunnel: w238 -> [w514]
            tunnel: w237 -> [w517]
            tunnel: [w527] -> w236
            tunnel: [w526] -> w235
            tunnel: w223 -> [w524]
            stop <- w528 stop-if-true
            # "DAQ Output (Start Last / End First)"
            n140 = local read "AO/DO SampRate"() -> (w508:dbl)
            n141 = Unbundle By Name(w524) -> ("piezo_command"=w518:dbl[], "alignment_command"=w519:dbl[])
            n142 = Reciprocal(x=w508) -> (1/x=w507:dbl)
            n143 = Array Size(array=w519) -> (size(s)=w509:i32)
            "N Samps 2 Write" <- w509
            n144 = Bundle By Name("Y"=w518, "dt"=w507) -> (→"Curr Piezo Cmd":waveform(dbl))  [unwired: 1 in]
            n145 = call <vilib>:"DAQmx Configure Output Buffer.vi"("task/channels in"=w511, "buffer size (in samples per channel)"=w509, "error in"=w510) -> ("task out"=w512:refnum<k21>, "error out"=w513:errorcluster)  [unwired: 11 in]
            n146 = call <vilib>:"DAQmx Configure Output Buffer.vi"("task/channels in"=w517, "buffer size (in samples per channel)"=w509, "error in"=w514) -> ("task out"=w516:refnum<k21>, "error out"=w515:errorcluster)  [unwired: 11 in]
            n147 = local read "Acquiring Frames"() -> (w530:bool)
            n148 = Multiply(x=w507, y=w509) -> (x*y=w506:dbl)
            n149 = Multiply(x=1.0, y=w506) -> (x*y=w504:dbl)
            n150 = call "analog2digital_wf_array.vi"("analog waveform"=w519) -> ("digital array"=w523:digitalwaveform[])  [unwired: 7 in, 3 out]
            n151 = case shown="True" w530 {
              tunnel: w513 -> [w534 w564]
              tunnel: w512 -> [w535 w565]
              tunnel: [w535 w567] -> w529
              tunnel: [w534 w566] -> w525
              tunnel: [FALSE ("Stop Input") TRUE ("Stop Input")] -> w520
              tunnel: w515 -> [w532 w562]
              tunnel: [w532 w559] -> w526
              tunnel: [w531 w560] -> w527
              tunnel: w516 -> [w531 w561]
              tunnel: w523 -> [_ w558]
              tunnel: w518 -> [_ w545]
              tunnel: w504 -> [_ w537]
              frame False {
              }
              frame True {
                n152 = call-poly <vilib>:"DAQmx Write.vi"("task/channels in"=w561, "auto start"=FALSE, "data"=w558, "error in"=w562) -> ("task out"=w548:refnum<k21>, "number of samples written per channel"=→"DO Samps Written":u32, "error out"=w549:errorcluster)  [unwired: 9 in]
                n153 = call-poly <vilib>:"DAQmx Write.vi"("task/channels in"=w565, "auto start"=FALSE, "data"=w545, "error in"=w564) -> ("task out"=w546:refnum<k21>, "number of samples written per channel"=→"AO Samps Written":u32, "error out"=w547:errorcluster)  [unwired: 9 in]
                n154 = flat-sequence {
                  tunnel: w549 -> [w573]
                  tunnel: w548 -> [w572]
                  tunnel: [w571] -> w557
                  tunnel: [w570] -> w556
                  tunnel: [w569] -> w555
                  tunnel: w547 -> [w569]
                  tunnel: w546 -> [w568]
                  tunnel: [w568] -> w554
                  tunnel: [w578] -> w536
                  tunnel: [w579] -> w538
                  tunnel: w557 -> [w579]
                  tunnel: w556 -> [w578]
                  tunnel: w555 -> [w577]
                  tunnel: [w576] -> w541
                  tunnel: [w575] -> w542
                  tunnel: w554 -> [w574]
                  frame #0 {
                    n155 = call <vilib>:"DAQmx Start Task.vi"("task/channels in"=w572, "error in"=w573) -> ("task out"=w571:refnum<k21>, "error out"=w570:errorcluster)  [unwired: 12 in]
                  }
                  frame #1 {
                    n156 = call <vilib>:"DAQmx Start Task.vi"("task/channels in"=w574, "error in"=w577) -> ("task out"=w575:refnum<k21>, "error out"=w576:errorcluster)  [unwired: 12 in]
                  }
                }
                n157 = call <vilib>:"DAQmx Wait Until Done.vi"("task/channels in"=w538, "timeout (sec)"=w537, "error in"=w536) -> ("task out"=w540:refnum<k21>, "error out"=w539:errorcluster)  [unwired: 11 in]
                n158 = call <vilib>:"DAQmx Wait Until Done.vi"("task/channels in"=w542, "timeout (sec)"=w537, "error in"=w541) -> ("task out"=w543:refnum<k21>, "error out"=w544:errorcluster)  [unwired: 11 in]
                n159 = call <vilib>:"DAQmx Stop Task.vi"("task/channels in"=w543, "error in"=w544) -> ("task out"=w567:refnum<k21>, "error out"=w566:errorcluster)  [unwired: 12 in]
                n160 = call <vilib>:"DAQmx Stop Task.vi"("task/channels in"=w540, "error in"=w539) -> ("task out"=w560:refnum<k21>, "error out"=w559:errorcluster)  [unwired: 12 in]
              }
            }
            n161 = Merge Errors(w525, w526) -> (w521:errorcluster)
            n162 = Or(x=w521, y=w520) -> (x .or. y?=w528:bool)
          }
          n163 = local read "AI/DI SampRate"() -> (w215:dbl)
          n164 = flat-sequence {
            tunnel: w269 -> [w287]
            tunnel: w232 -> [w286]
            tunnel: w214 -> [w288]
            tunnel: [w287] -> w231
            tunnel: [w286] -> w230
            tunnel: [w290] -> w229
            tunnel: [w289] -> w228
            tunnel: [w295] -> w233
            tunnel: [w296] -> w234
            tunnel: [w293] -> w278
            tunnel: [w294] -> w279
            tunnel: w231 -> [w291]
            tunnel: w230 -> [w292]
            tunnel: w229 -> [w296]
            tunnel: w228 -> [w295]
            frame #0 {
              # "DI"
              n165 = call <vilib>:"DAQmx Start Task.vi"("task/channels in"=w288, "error in"=w286) -> ("task out"=w289:refnum<k21>, "error out"=w290:errorcluster)  [unwired: 12 in]
            }
            frame #1 {
              # "AI"
              n166 = call <vilib>:"DAQmx Start Task.vi"("task/channels in"=w291, "error in"=w292) -> ("task out"=w294:refnum<k21>, "error out"=w293:errorcluster)  [unwired: 12 in]
            }
          }
          n167 = call "make_recording_h5_files.vi"("output rate"=w205, "input rate"=w206, "write/append size"=w215, "Path"=w247) -> ("error out"=w246:errorcluster, "output cluster"=w219:T7, "ref out"=w244:T8)  [unwired: 5 in]
          n168 = while {
            tunnel: w246 -> [w587]
            tunnel: [w608] -> w277
            shift-right: [w620] -> w275
            shift-left: w279 -> [w626]
            shift-right: [w619] -> w274
            shift-left: w278 -> [w625]
            tunnel: [w618] -> w245
            tunnel: w244 -> [w618]
            shift-right: [w613] -> w226
            shift-left: w234 -> [w615]
            shift-right: [w614] -> w227
            shift-left: w233 -> [w616]
            tunnel: w215 -> [w611]
            tunnel: w219 -> [w610]
            tunnel: w204 -> [w586]
            stop <- w617 stop-if-true
            # "Sensor Ch"
            # "Piezo Ch"
            # "700b\nSecondary"
            # "700b\nPrimary"
            # "align sig"
            # "700b\nCommand\nDummy Ch."
            # "700b \nMode\nDummy Ch."
            # "End when frame acquisition stops"
            # "DAQ Input (Start First / End Last)"
            n169 = Unbundle By Name(w610) -> ("mc700b_primary"=w588:i32, "mc700b_secondary"=w589:i32, "piezo_cmd"=w590:i32, "piezo_sensor"=w591:i32, "cam_trig_1"=w582:i32, "cam_trig_2"=w581:i32, "alignment_cmd"=w580:i32)  [unwired: 2 out]
            n170 = call-poly <vilib>:"DAQmx Read.vi"("task/channels in"=w626, "number of samples per channel"=w611, "error in"=w625) -> ("task out"=w620:refnum<k21>, "data"=w593:waveform(dbl)[], "error out"=w619:errorcluster)  [unwired: 10 in]
            "DAC Input" <- w593
            n171 = call-poly <vilib>:"DAQmx Read.vi"("task/channels in"=w616, "number of samples per channel"=w611, "error in"=w615) -> ("task out"=w614:refnum<k21>, "data"=w585:u32[][], "error out"=w613:errorcluster)  [unwired: 10 in]
            n172 = Index Array(array=w593, index=2) -> (element=w607:waveform(dbl))
            n173 = Index Array(array=w593, index=3) -> (element=w605:waveform(dbl))
            n174 = Index Array(array=w593, index=0) -> (element=w624:waveform(dbl))
            n175 = Index Array(array=w593, index=1) -> (element=w622:waveform(dbl))
            n176 = Index Array(array=w585, index (row)=2 ("index")) -> (element=w609:u32[])  [unwired: 1 in]
            n177 = Unbundle By Name(w607) -> ("Y"=w603:dbl[])
            n178 = Unbundle By Name(w605) -> ("Y"=w602:dbl[])
            n179 = Unbundle By Name(w624) -> ()  [unwired: 1 out]
            n180 = Unbundle By Name(w622) -> ()  [unwired: 1 out]
            n181 = call "append_h5_dataset.vi"() -> ()  [unwired: 11 in, 1 out]
            n182 = call "append_h5_dataset.vi"() -> ()  [unwired: 11 in, 1 out]
            n183 = call "append_h5_dataset.vi"("error in (no error)"=w587, "Data"=w603, "dset in"=w588) -> ("error out"=w601:errorcluster)  [unwired: 8 in]
            n184 = call "append_h5_dataset.vi"("error in (no error)"=w601, "Data"=w602, "dset in"=w589) -> ("error out"=w592:errorcluster)  [unwired: 8 in]
            n185 = Index Array(array=w593, index=4) -> (element=w600:waveform(dbl))
            n186 = Index Array(array=w593, index=5) -> (element=w598:waveform(dbl))
            n187 = Unbundle By Name(w600) -> ("Y"=w596:dbl[])
            n188 = Unbundle By Name(w598) -> ("Y"=w595:dbl[])
            n189 = local read "Stop Input"() -> (w617:bool)
            n190 = call "append_h5_dataset.vi"("error in (no error)"=w592, "Data"=w596, "dset in"=w590) -> ("error out"=w594:errorcluster)  [unwired: 8 in]
            n191 = call "append_h5_dataset.vi"("error in (no error)"=w594, "Data"=w595, "dset in"=w591) -> ("error out"=w584:errorcluster)  [unwired: 8 in]
            n192 = case shown="True" w586 {
              tunnel: w585 -> [_ w633]
              tunnel: w584 -> [w627 w632]
              tunnel: [w627 w630] -> w583
              tunnel: w582 -> [_ w629]
              tunnel: w581 -> [_ w628]
              frame False {
              }
              frame True {
                # "cam trig 2"
                # "cam trig 1"
                n193 = Index Array(array=w633, index (row)=1 ("index")) -> (element=w634:u32[])  [unwired: 1 in]
                n194 = Index Array(array=w633, index (row)=0 ("index")) -> (element=w636:u32[])  [unwired: 1 in]
                n195 = call "append_h5_dataset.vi"("error in (no error)"=w632, "Data"=w636, "dset in"=w629) -> ("error out"=w631:errorcluster)  [unwired: 8 in]
                n196 = call "append_h5_dataset.vi"("error in (no error)"=w631, "Data"=w634, "dset in"=w628) -> ("error out"=w630:errorcluster)  [unwired: 8 in]
              }
            }
            n197 = call "append_h5_dataset.vi"("error in (no error)"=w583, "Data"=w609, "dset in"=w580) -> ("error out"=w608:errorcluster)  [unwired: 8 in]
          }
          n198 = call <vilib>:"DAQmx Stop Task.vi"("task/channels in"=w275, "error in"=w274) -> ("task out"=w270:refnum<k21>, "error out"=w271:errorcluster)  [unwired: 12 in]
          n199 = call <vilib>:"H5Fclose.vi"("error in (no error)"=w277, "ref"=w245) -> ("error out"=w276:errorcluster)  [unwired: 9 in]
          n200 = call <vilib>:"DAQmx Stop Task.vi"("task/channels in"=w227, "error in"=w226) -> ("task out"=w225:refnum<k21>, "error out"=w224:errorcluster)  [unwired: 12 in]
        }
      }
    }
    frame Error {
    }
  }
  n201 = call <vilib>:"DAQmx Clear Task.vi"("task in"=w43, "error in"=w9) -> ("error out"=w41:errorcluster)  [unwired: 13 in]
  n202 = call <vilib>:"DAQmx Clear Task.vi"("task in"=w33, "error in"=w34) -> ("error out"=w32:errorcluster)  [unwired: 13 in]
  n203 = call <userlib>:"tm_closecamera.vi"("error in (no error)"=w36, "Handle in"=w35) -> ("error out"=w44:errorcluster)  [unwired: 9 in]
  n204 = call <vilib>:"DAQmx Clear Task.vi"("task in"=w18, "error in"=w17) -> ("error out"=w16:errorcluster)  [unwired: 13 in]
  n205 = call <vilib>:"DAQmx Stop Task.vi"("task/channels in"=w39, "error in"=w40) -> ("task out"=w46:refnum<k21>, "error out"=w45:errorcluster)  [unwired: 12 in]
  n206 = call <vilib>:"DAQmx Clear Task.vi"("task in"=w19, "error in"=w20) -> ("error out"=w21:errorcluster)  [unwired: 13 in]
  n207 = call <userlib>:"tm_deinitialize.vi"("error in (no error)"=w44) -> ("error out"=w37:errorcluster)  [unwired: 10 in]
  n208 = call <vilib>:"DAQmx Clear Task.vi"("task in"=w46, "error in"=w45) -> ("error out"=w38:errorcluster)  [unwired: 13 in]
  n209 = Merge Errors(w15, w16, w21, w37, w38, w42, w41, w32, w29) -> (→"error out":errorcluster)
